vi "Find Ideal Range.vi"(8 "error in":errorcluster, 11 "3300 in":refnum<class "3300.lvclass">) -> (0 "error out":errorcluster, 2 "Ideal Range":cluster{"Low":dbl, "High":dbl}, 3 "3300 out":refnum<class "3300.lvclass">)   [LabVIEW 2019, in "3300.lvlib" / "3300.lvclass"]
uses:
  Library/3300.lvclass
  C:/Users/Public/Documents/Development/builds/Instruments/Electronic Load.lvlibp/Library/Electronic Load.lvclass
  Module Support/Access Module Ranges.vi
  builds/Instruments/Electronic Load.lvlibp/Accessors/Trigger/Read Pulse Initial.vi
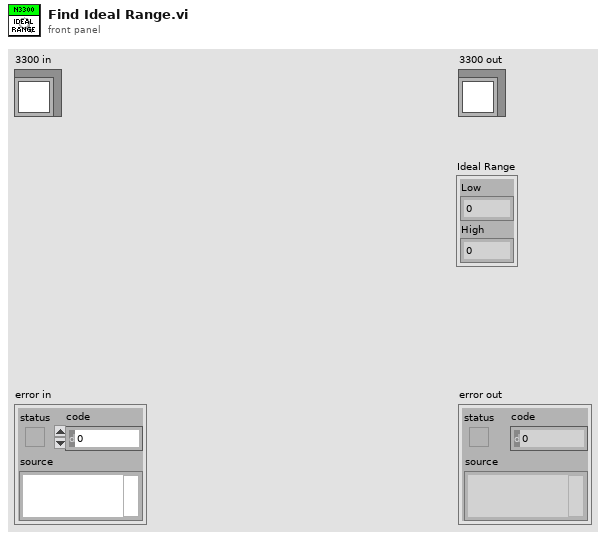
[diagram p1: front panel]
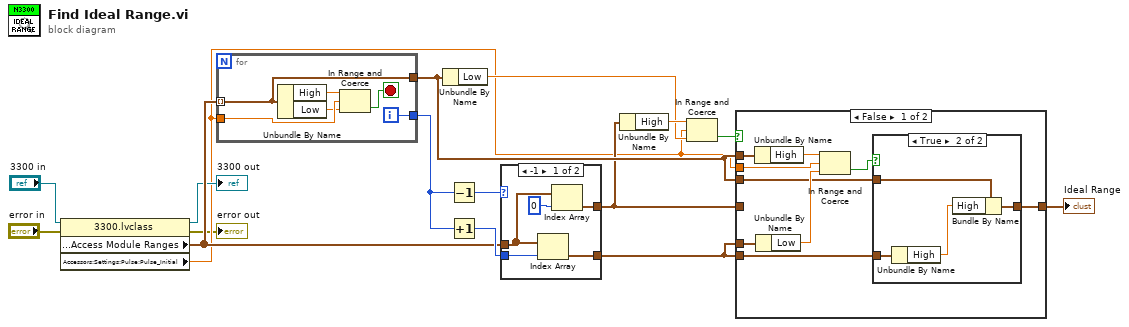
[diagram p0: block diagram]
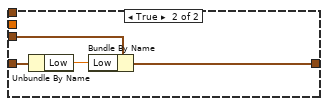
[diagram p3: hidden frame]
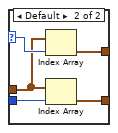
[diagram p4: hidden frame]
diagram:
  n1 = property class="3300.lvclass"(reference="3300 in", error in="error in") -> (reference out=→"3300 out":refnum<class "3300.lvclass">, error out=→"error out":errorcluster, "Private:Accessors:Access Module Ranges"=w5:cluster{"Low":dbl, "High":dbl}[], "Accessors:Settings:Pulse:Pulse_Initial"=w2:dbl)
  n2 = for {
    tunnel: w5 -> [w19] mode=indexing
    tunnel: w2 -> [w21]
    tunnel: [w22] -> w8
    tunnel: [w19] -> w14
    i -> [w22]
    stop <- w20 stop-if-true
    n3 = Unbundle By Name(w19) -> ("High"=w17:dbl, "Low"=w18:dbl)
    n4 = In Range and Coerce(upper limit=w17, x=w21, lower limit=w18) -> (In Range?=w20:bool)  [unwired: 1 out]
  }
  n5 = Unbundle By Name(w14) -> ("Low"=w10:dbl)
  n6 = Decrement(x=w8) -> (x-1=w7:i32)
  n7 = Increment(x=w8) -> (x+1=w9:i32)
  n8 = case shown="-1" w7 {
    selector: w7 -> [_ w30]
    tunnel: w5 -> [w25 w29]
    tunnel: [w26 w32] -> w13
    tunnel: [w24 w31] -> w16
    tunnel: w9 -> [w23 w28]
    frame -1 {
      n9 = Index Array(array=w25, index=w23) -> (element=w24:cluster{"Low":dbl, "High":dbl})
      n10 = Index Array(array=w25, index=0) -> (element=w26:cluster{"Low":dbl, "High":dbl})
    }
    frame Default {
      n11 = Index Array(array=w29, index=w30) -> (element=w32:cluster{"Low":dbl, "High":dbl})
      n12 = Index Array(array=w29, index=w28) -> (element=w31:cluster{"Low":dbl, "High":dbl})
    }
  }
  n13 = Unbundle By Name(w13) -> ("High"=w11:dbl)
  n14 = In Range and Coerce(upper limit=w11, x=w2, lower limit=w10) -> (In Range?=w12:bool)  [unwired: 1 out]
  n15 = case shown="False" w12 {
    tunnel: w13 -> [_ w48]
    tunnel: w14 -> [w41 _]
    tunnel: w16 -> [w39 _]
    tunnel: w2 -> [w37 _]
    tunnel: w14 -> [w35 w50]
    tunnel: [w34 w49] -> w15
    tunnel: w16 -> [w33 _]
    frame False {
      n16 = Unbundle By Name(w41) -> ("High"=w40:dbl)
      n17 = Unbundle By Name(w39) -> ("Low"=w38:dbl)
      n18 = In Range and Coerce(upper limit=w40, x=w37, lower limit=w38) -> (In Range?=w36:bool)  [unwired: 1 out]
      n19 = case shown="True" w36 {
        tunnel: w35 -> [w42 w46]
        tunnel: [w42 w44] -> w34
        tunnel: w33 -> [_ w45]
        frame False {
        }
        frame True {
          n20 = Unbundle By Name(w45) -> ("High"=w43:dbl)
          n21 = Bundle By Name(cluster=w46, "High"=w43) -> (w44:cluster{"Low":dbl, "High":dbl})
        }
      }
    }
    frame True {
      n22 = Unbundle By Name(w48) -> ("Low"=w47:dbl)
      n23 = Bundle By Name(cluster=w50, "Low"=w47) -> (w49:cluster{"Low":dbl, "High":dbl})
    }
  }
  "Ideal Range" <- w15
